vi "Find_Max_Value.vi"(3 "Mode":T6, 5 "Traverse line In":T1 {"Row Duration (mins)" format="%#.1f"; "Row No" min=0; "Trace Gas Concentration (%)" min=0.0 format="%#.2f"; "Emission Rate (l/min)" format="%#.2f"; "Tunnel Speed" format="%#.2f"; "Start X" format="%#.2f"; "Start Y" format="%#.2f"; "Start Z" format="%#.2f"; "End X" format="%#.2f"; "End Y" format="%#.2f"; "End Z" format="%#.2f"; "Averaging time (min)" min=0.0 format="%#.2f"}) -> (0 "Error Message":string, 1 "Status":T5, 2 "Traverse line Out":T1 {"Row Duration (mins)" format="%#.1f"; "Row No" min=0; "Trace Gas Concentration (%)" min=0.0 format="%#.2f"; "Emission Rate (l/min)" format="%#.2f"; "Tunnel Speed" format="%#.2f"; "Start X" format="%#.2f"; "Start Y" format="%#.2f"; "Start Z" format="%#.2f"; "End X" format="%#.2f"; "End Y" format="%#.2f"; "End Z" format="%#.2f"; "Averaging time (min)" min=0.0 format="%#.2f"})   [LabVIEW 2011]
uses:
  Controls/User_Specific_mode.ctl
  Gen Trav/Multi_Run_Status.ctl
  Gen Trav/Route mapping/Axis.ctl
  Gen Trav/Traverse_cluster.ctl
  Gen Trav/Spacing.ctl
  Controls/Multi_run_mode.ctl
  Controls/Tunnel_Coordinates.ctl
  Gen Trav/Trav_mode.ctl
  Controls/Save_Data.ctl
  Controls/Setup.ctl
  Globals/Meas_global.vi
panel:
  out "Measured Instrument":string
  out "Value to Measure":string
  in  "Channel to Measure":i32
  in  "Simulate?":bool
  in  "Picture Filename":path
  out "vi reference":refnum<vi>
  in  "Search Step (mm)":dbl=1.0
  out "Value at Maxima":dbl
  in  "Starting Position":dbl[](array[numeric]) format="%.1f"
  in  "stop":bool
  out "Message":string
  out "Y":i32
  out "X":i32
  out "Array 2":dbl[](array[numeric]) format="%.4f"
  out "Measured Points":dbl[][](array[numeric]) format="%.2f"
  out "Current Value":dbl format="%.2f"
  out "Current Index":i32
  out "Array":i32[][](array[numeric])
  out "Measurement":dbl[][](graph)
  out "Found Maxima?":bool
  out "Meas maxima":dbl[](array[numeric]) format="%.1f"
  out "Present Position":dbl[](array[numeric])
  out "Profile":dbl[][](array[numeric]) format="%.2f"
  in  "Fixed Axis":T4
  # "X           Y            Z"
  # "Start"
  # "End"
  # "X           Y            Z"
  # "Start"
  # "End"
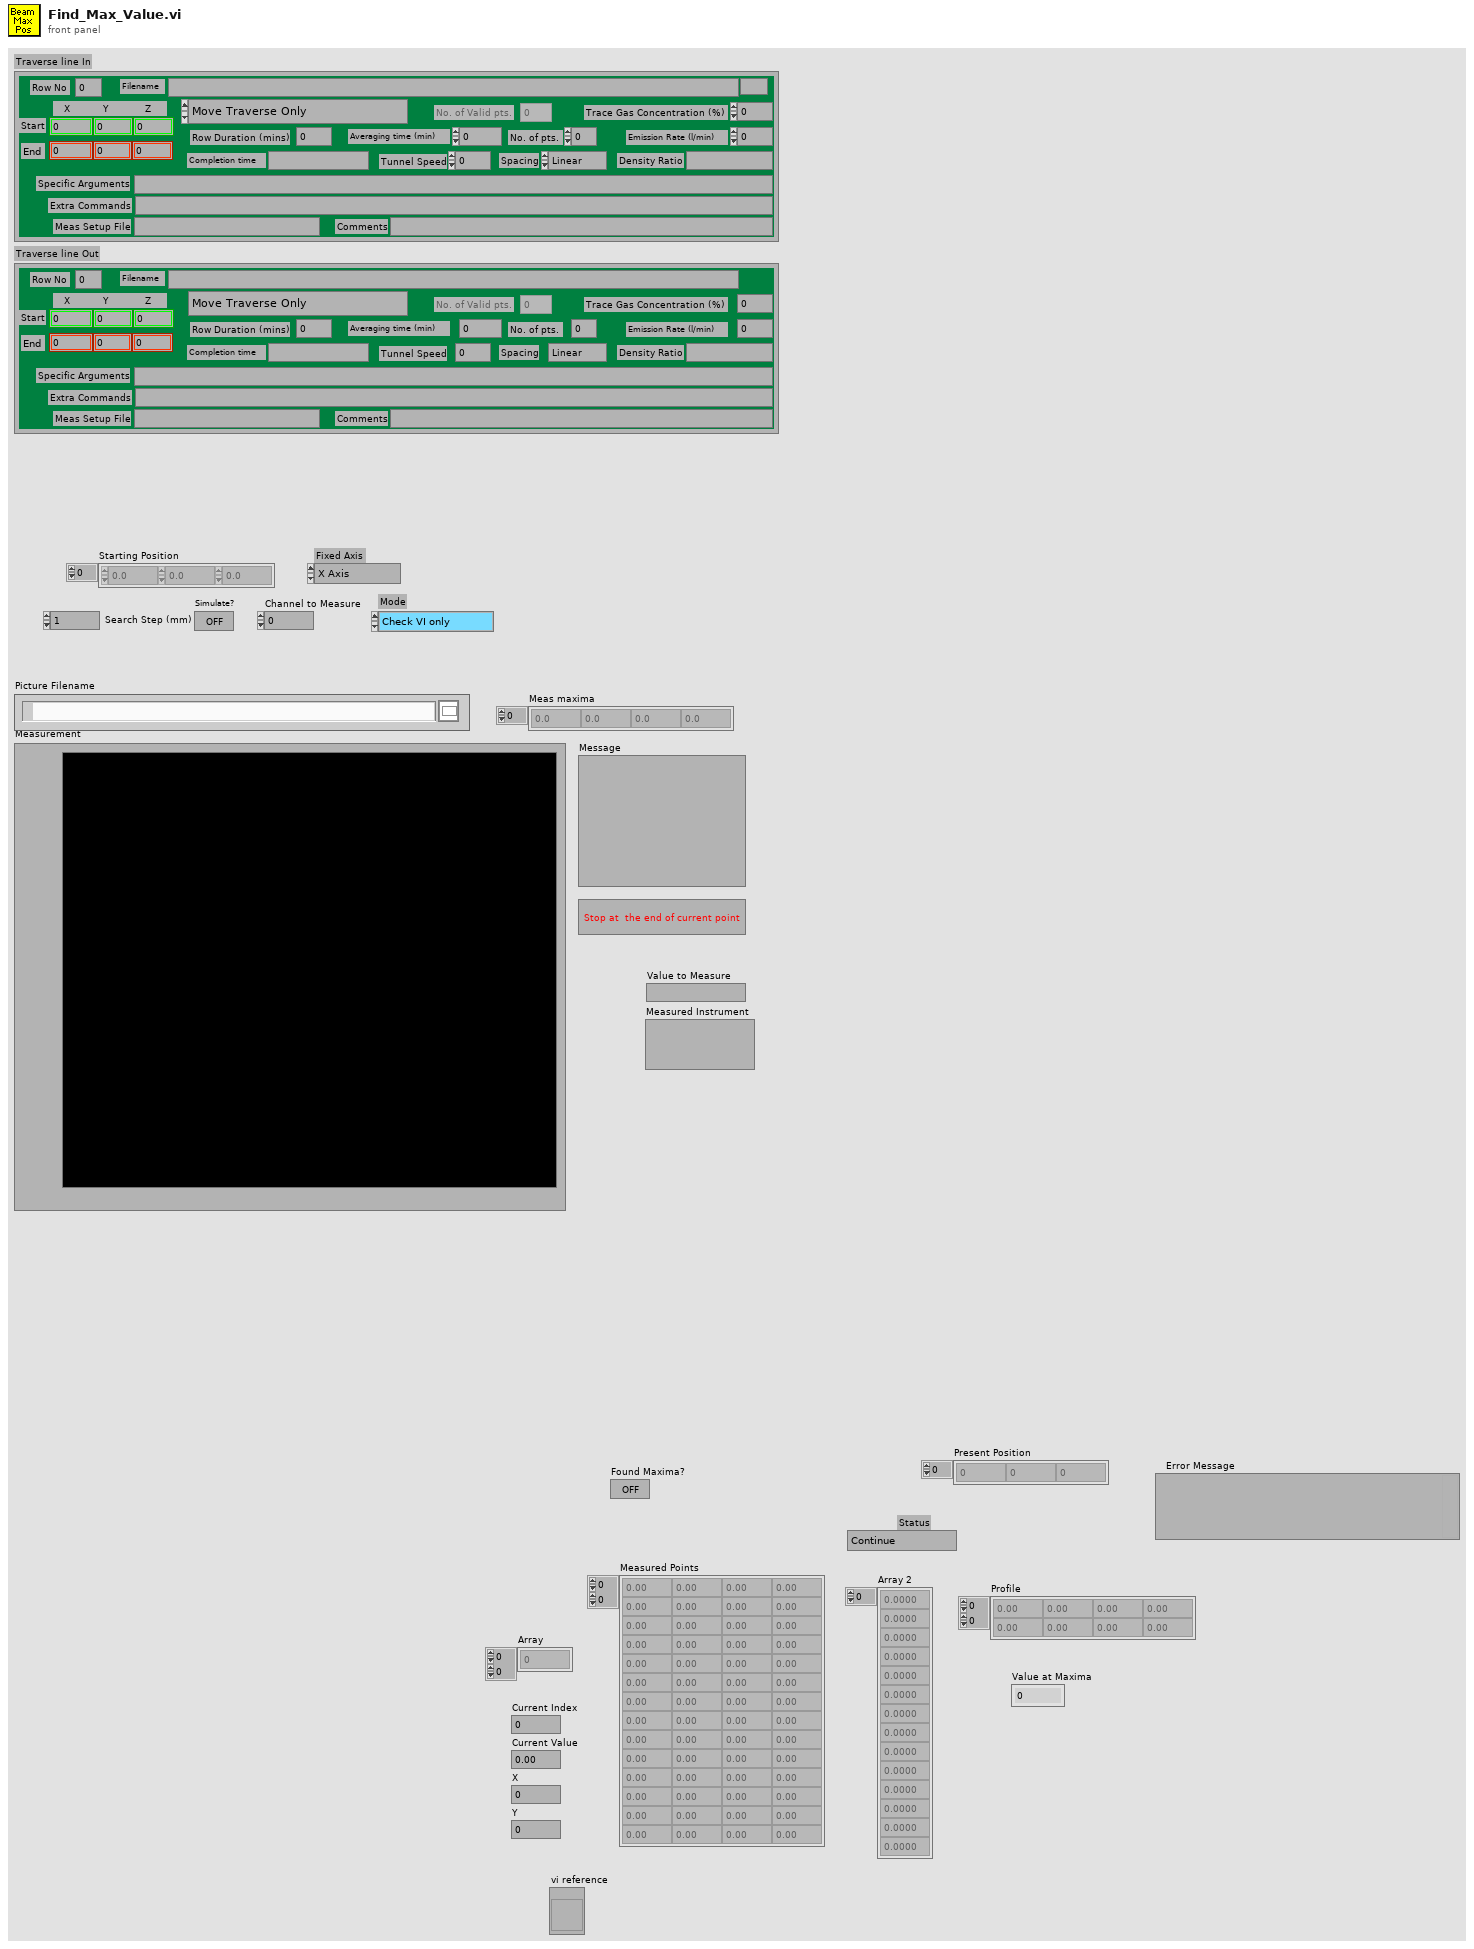
[diagram p1: front panel]
types:
  T1 = typedef "Traverse_cluster.ctl" = cluster{"Start X":dbl, "Start Y":dbl, "Start Z":dbl, "End X":dbl, "End Y":dbl, "End Z":dbl, "No. of pts.":i32, "Spacing":T2, "Filename":path, "Tunnel Speed":dbl, "Averaging time (min)":dbl, "Extra Commands":string, "Specific Arguments":string, "Emission Rate (l/min)":dbl, "Trace Gas Concentration (%)":dbl, "Density Ratio":string, "Comments":string, "Row No":i32, "Row Type Selector":T3, "Completion time":string, "Row Duration (mins)":dbl, "No. of Valid pts.":i32, "Meas Setup File":string}
  T2 = typedef "Spacing.ctl" = enum16{"Linear", "Log", "Gauss", "Specified", "N/A"}
  T3 = typedef "Multi_run_mode.ctl" = enum16{"Move Traverse Only", "Set Tunnel Speed Only", "Set Source Only", "Set Measurement Conditions", "Single Measurement", "Vertical Profile", "Lateral Profile", "Longitudinal Profile", "Explore Volume", "Multi-Axis Profile", "Auto Calibrate", "Meas Fast FID Bkgnd", "Check Beam Power", "Scanning Valve Measurement", "Run VI Named:", "Set ADAM Ch", "Wait (minutes)", "Send Message", "Synchronize With:", "Fall Back to this Row", "Turn Off Row Repeating", "Blank Row", "Traverse 3D Volume"}
  T4 = typedef "Axis.ctl" = enum16{"X Axis", "X Axis -ve", "Y Axis", "Y Axis -ve", "Z Axis", "Z Axis -ve"}
  T5 = typedef "Multi_Run_Status.ctl" = enum16{"Continue", "Jump to Next Point", "Jump to Next Row", "Jump To Fall Back", "Terminate Run"}
  T6 = typedef "User_Specific_mode.ctl" = enum16{"Check VI only", "Run VI"}
  T7 = typedef "Tunnel_Coordinates.ctl" = enum16{"Work in Tunnel Coordinates", "Work in Model Coordinates"}
  T8 = typedef "Trav_mode.ctl" = enum16{"Move traverse", "Read traverse position", "Teach Position"}
  T9 = cluster{"Status":enum16{"Continue", "Jump to Next Point", "Jump to Next Row", "Jump To Fall Back", "Terminate Run"}, "Error Type":string, "Error Description":string}
  T10 = typedef "Save_Data.ctl" = enum16{"Save No Data", "Save Data"}
  T11 = typedef "Setup.ctl" = enum16{"Run Program", "Show Setup", "Save Current Setup", "Setup Front Panel"}
  T12 = typedef "Status_Cluster.ctl" = cluster{"Status":T5, "Error Type":string, "Error Description":string}
  T13 = typedef "Analysis_info_cluster.ctl" = cluster{"Colour":u32, "Inst type":T14, "Inst name":string, "Symbol":string, "Code name":string, "Extra Info":string, "Inst Array":T15, "Extra Titles":string[], "Extra Values":string[], "U":dbl, "u^2":dbl, "u^3":dbl, "u^4":dbl, "Skew_u":dbl, "Kurt_u":dbl, "Sd Error in Mean":dbl, "% u'/U":dbl, "X":dbl, "Y":dbl, "Z":dbl, "Timescale integral to 25%":dbl, "Sd Error in Variance":dbl, "Calib File":path, "Calib Constants":dbl[], "Output Position":bool, "Full Stats":bool, "Av Sampling Rate":dbl, "Av No of Samples":dbl, "Total Meas Time (s)":dbl, "ADAM Ch Name":string}
  T14 = typedef "Inst_type.ctl" = enum16{"Propeller anemometer", "Raw voltage", "Pressure Transducer", "Pitot-static tube", "Preston tube", "Hot wire", "Cross wire 1", "Cross wire 2", "Generic Linear", "Generic Polynomial", "Generic BackPoly", "Fast FID", "Thermocouple", "Cold wire", "Pulsed Wire", "LDA Vel", "LDA Tran time", "LDA Arr time"}
  T15 = typedef "Instrument_Array.ctl" = enum16{"PWA", "LDA", "Analogue"}
  T16 = typedef "Correlation_cluster1.ctl" = cluster{"U inst":string, "uw":dbl, "u^2w":dbl, "uw^2":dbl, "uw/u'w'":dbl, "W inst":string, "uw^3":dbl, "u^3w":dbl, "u^2w^2":dbl, "Index U":i32, "Index W":i32}
  T17 = typedef "LVRectTypeDef.ctl" = cluster{"left":i16, "top":i16, "right":i16, "bottom":i16}
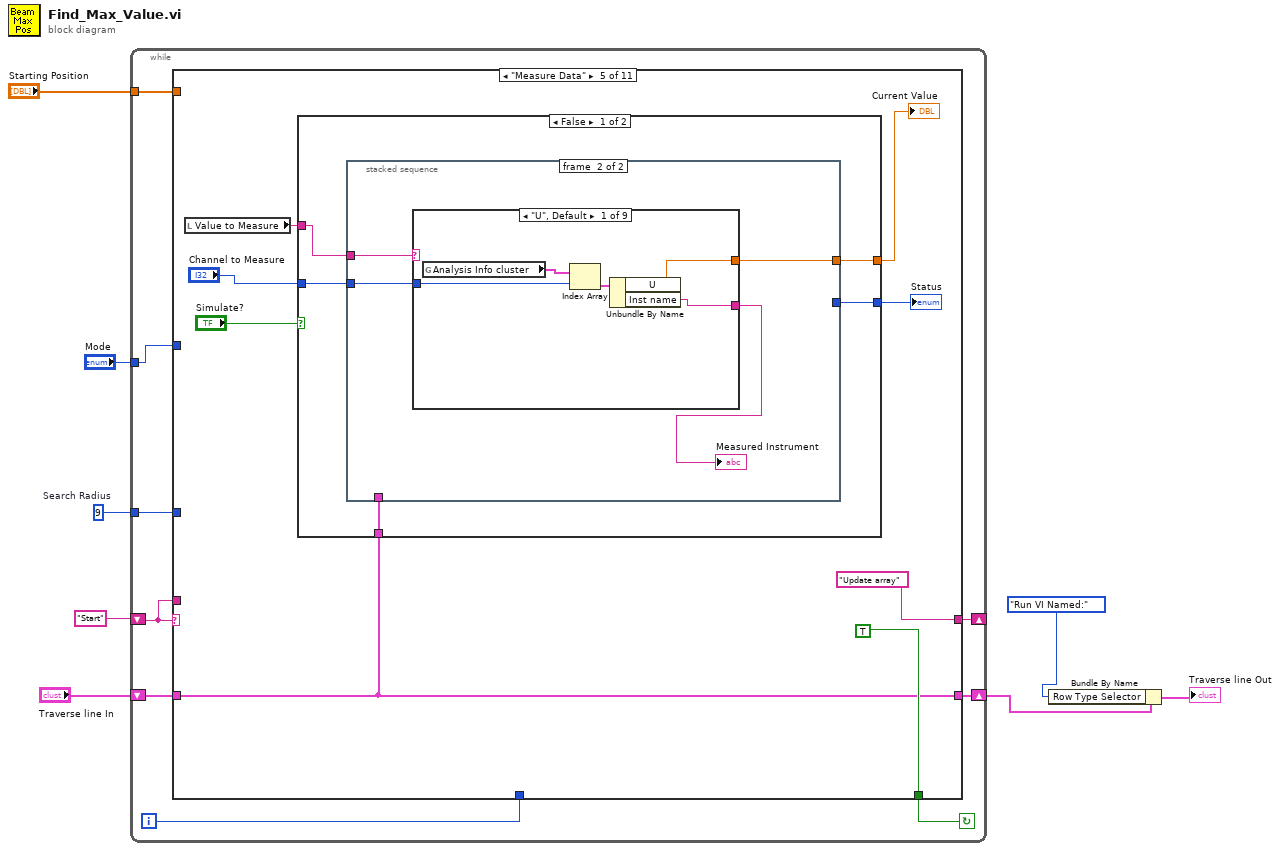
[diagram p0: block diagram]
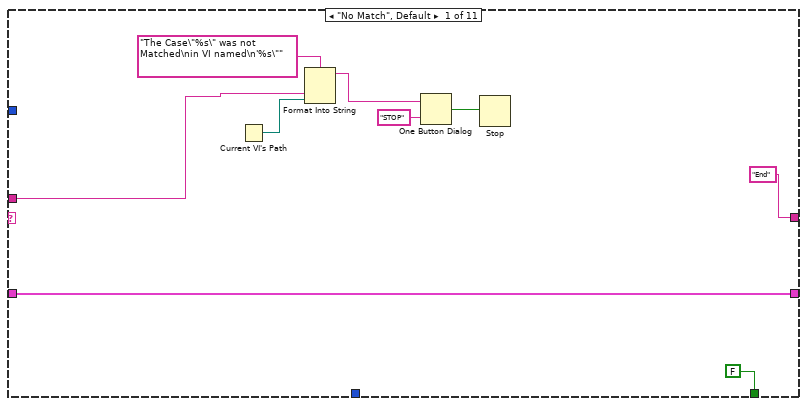
[diagram p2: hidden frame]
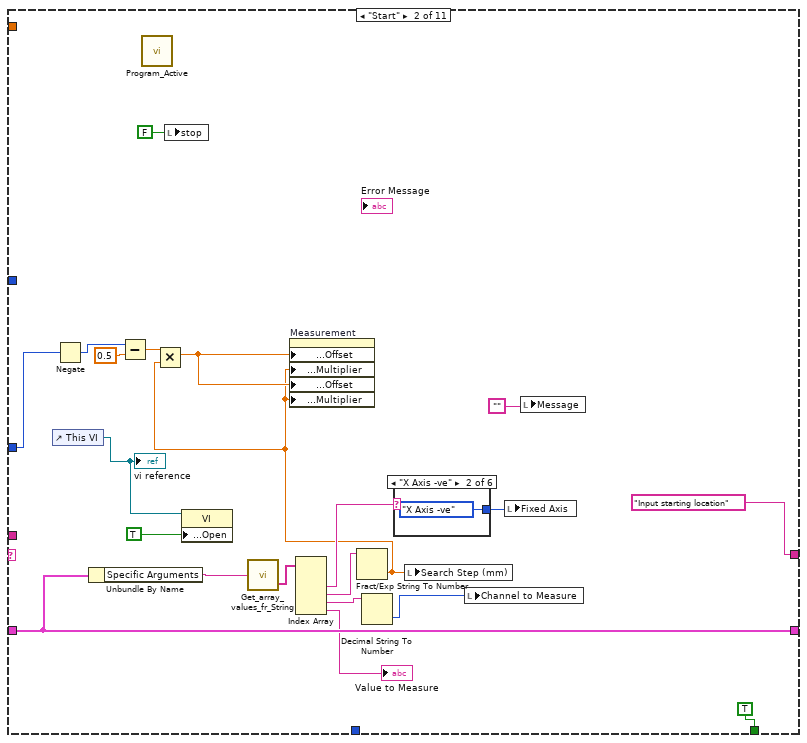
[diagram p3: hidden frame]
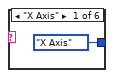
[diagram p4: hidden frame]
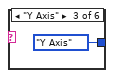
[diagram p5: hidden frame]
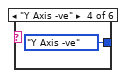
[diagram p6: hidden frame]
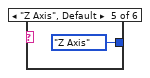
[diagram p7: hidden frame]
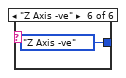
[diagram p8: hidden frame]
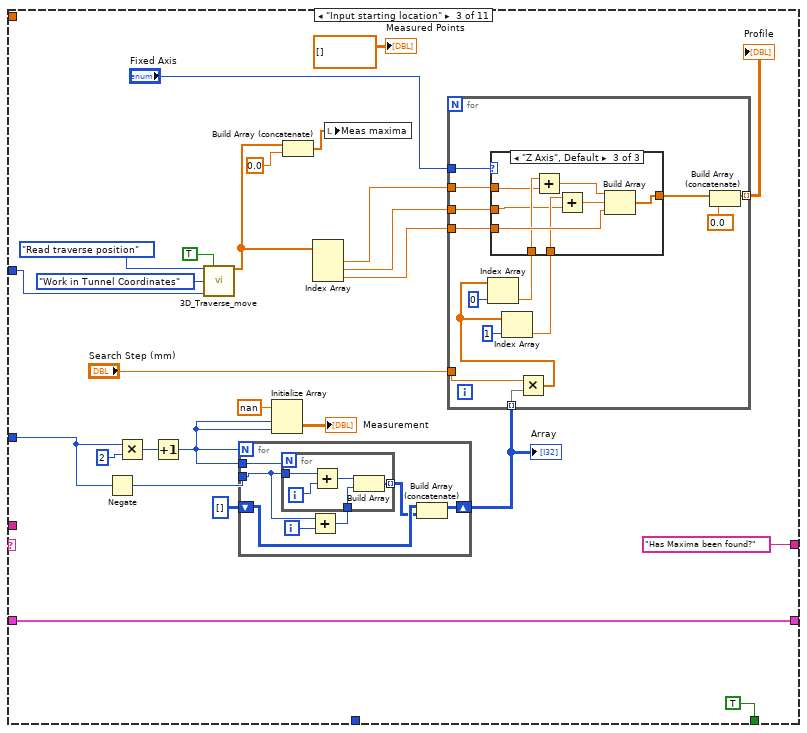
[diagram p9: hidden frame]
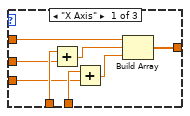
[diagram p10: hidden frame]
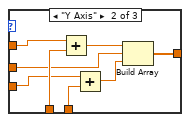
[diagram p11: hidden frame]
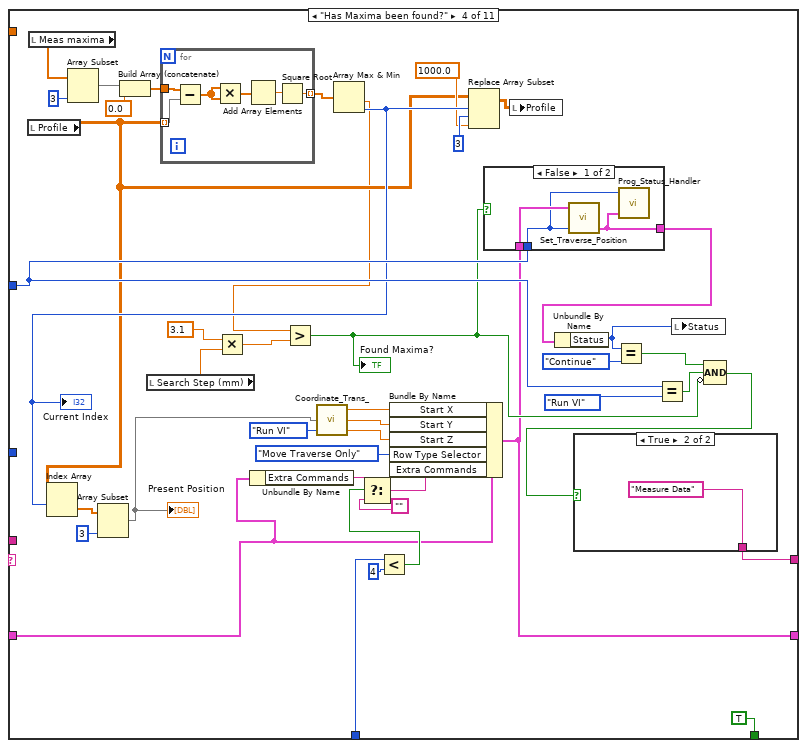
[diagram p12: hidden frame]
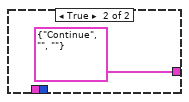
[diagram p13: hidden frame]
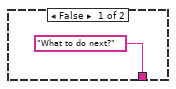
[diagram p14: hidden frame]
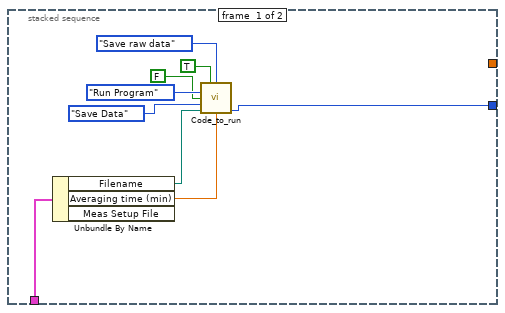
[diagram p15: hidden frame]
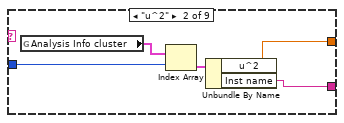
[diagram p16: hidden frame]
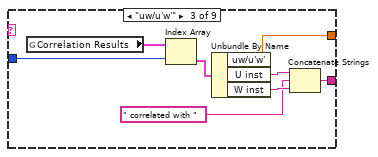
[diagram p17: hidden frame]
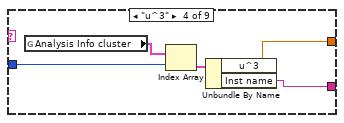
[diagram p18: hidden frame]
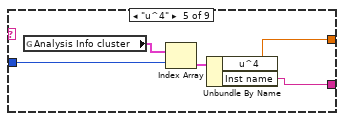
[diagram p19: hidden frame]
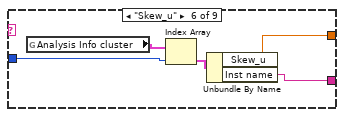
[diagram p20: hidden frame]
diagram:
  w7 = 9  # Search Radius
  n1 = while {
    tunnel: "Mode" -> [w15]
    shift-left: "Start" -> [w11]
    shift-right: [w16] -> _
    tunnel: w7 -> [w14]
    tunnel: "Starting Position" -> [w13]
    shift-right: [w9] -> w2
    shift-left: "Traverse line In" -> [w10]
    i -> [w12]
    stop <- w17 continue-if-true
    n2 = case shown="\"Measure Data\"" w11 {
      tunnel: w15 -> [_ _ w62 w167 _ _ _ w335 _ _ _]
      tunnel: [FALSE TRUE TRUE TRUE TRUE TRUE TRUE w329 TRUE TRUE FALSE] -> w17
      tunnel: ["End" "Input starting location" "Has Maxima been found?" w148 "Update array" "Calculate new maxima position" "What to do next?" w332 "Log Front Panel" "Get Interp Location" "End"] -> w16
      tunnel: w14 -> [_ w44 w69 _ _ w269 w289 _ _ _ _]
      tunnel: w13 -> [_ _ _ _ _ _ _ _ w355 _ _]
      tunnel: w12 -> [_ _ _ w134 _ _ _ _ _ _ _]
      tunnel: w11 -> [w21 _ _ _ _ _ _ _ _ _ _]
      tunnel: w10 -> [w18 w36 w64 w132 w186 w264 w282 w328 w343 w402 w417]
      tunnel: [w18 w36 w64 w131 w186 w264 w282 w328 w343 w402 w417] -> w9
      frame "No Match", Default {
        n3 = Current VI's Path() -> (path=w26:path)
        n4 = Format Into String(format string="The Case\"%s\" was not Matched\nin VI named\n'%s\"" ("Format String"), w21, w26) -> (resulting string=w23:string)  [unwired: 2 in, 1 out]
        n5 = One Button Dialog(message=w23, button name ("OK")="STOP") -> (true=w25:bool)
        n6 = Stop(stop? (T)=w25) -> ()
      }
      frame "Start" {
        n7 = control-ref of="This VI"() -> (w37:refnum<vi>)
        "vi reference" <- w37
        n8 = Negate(x=w44) -> (-x=w41:i32)
        n9 = Unbundle By Name(w36) -> ("Specific Arguments"=w35:string)
        n10 = Subtract(x=w41, y=0.5) -> (x-y=w42:dbl)
        n11 = call "Program_Active.vi"() -> ()  [unwired: 1 in]
        n12 = local write "stop"(FALSE ("stop")) -> ()
        n13 = property class="VI"(reference=w37, "Front Panel Window:Open"=TRUE) -> ()  [unwired: 1 in, 2 out]
        n14 = call "Get_array_values_fr_String.vi"("String Value"=w35) -> ("String array"=w34:string[])  [unwired: 1 out]
        n15 = Index Array(array=w34) -> (element #2=w33:string, element #3=w31:string, element #4=w29:string, element #5=→"Value to Measure":string)  [unwired: 5 in, 1 out]
        n16 = Fract/Exp String To Number(string=w31) -> (number=w30:dbl)  [unwired: 3 in, 1 out]
        n17 = Multiply(x=w42, y=w30) -> (x*y=w43:dbl)
        n18 = property on="Measurement" class="IntGraph (strict)"("X Scale.Offset and Multiplier:Offset"=w43, "X Scale.Offset and Multiplier:Multiplier"=w30, "Y Scale.Offset and Multiplier:Offset"=w43, "Y Scale.Offset and Multiplier:Multiplier"=w30) -> ()  [unwired: 2 in, 2 out]
        n19 = Decimal String To Number(string=w29) -> (number=w28:i32)  [unwired: 2 in, 1 out]
        n20 = case shown="\"X Axis -ve\"" w33 {
          tunnel: [Axis."X Axis" ("Fixed Axis") Axis."X Axis -ve" ("Fixed Axis") Axis."Y Axis" ("Fixed Axis") Axis."Y Axis -ve" ("Fixed Axis") Axis."Z Axis" ("Fixed Axis") Axis."Z Axis -ve" ("Fixed Axis")] -> w32
          frame "X Axis" {
          }
          frame "X Axis -ve" {
          }
          frame "Y Axis" {
          }
          frame "Y Axis -ve" {
          }
          frame "Z Axis", Default {
          }
          frame "Z Axis -ve" {
          }
        }
        n21 = local write "Search Step (mm)"(w30) -> ()
        n22 = local write "Channel to Measure"(w28) -> ()
        n23 = local write "Fixed Axis"(w32) -> ()
        n24 = local write "Message"("") -> ()
      }
      frame "Input starting location" {
        n25 = Negate(x=w69) -> (-x=w70:i32)
        n26 = Multiply(x=w69, y=2) -> (x*y=w67:i32)
        n27 = Increment(x=w67) -> (x+1=w66:i32)
        n28 = call "3D_Traverse_move.vi"("Mode"=Trav_mode."Read traverse position", "Route Checking?"=TRUE, "Work in Tunnel Coordinates"=Tunnel_Coordinates."Work in Tunnel Coordinates", "Simulate/Run"=w62) -> ("Trav Position achieved"=w59:dbl[])  [unwired: 9 in, 2 out]
        n29 = for {
          N: w66 -> [_]
          tunnel: w66 -> [w86]
          tunnel: w70 -> [w84]
          shift-right: [w80] -> w74
          shift-left: i32[][] [] -> [w82]
          i -> [w85]
          n30 = Add(x=w84, y=w85) -> (x+y=w83:i32)
          n31 = for {
            N: w86 -> [_]
            tunnel: w84 -> [w90]
            tunnel: w83 -> [w88]
            tunnel: [w87] -> w81 mode=indexing
            i -> [w91]
            n32 = Add(x=w90, y=w91) -> (x+y=w89:i32)
            n33 = Build Array(w89, w88) -> (w87:i32[])
          }
          n34 = Build Array (concatenate)(w82, w81) -> (w80:i32[][])
        }
        "Array" <- w74
        n35 = Initialize Array(nan, w66, w66) -> (→"Measurement":dbl[][])
        n36 = Build Array (concatenate)(w59, 0.0 ("Numeric")) -> (w76:dbl[])
        n37 = Index Array(array=w59) -> (element #1=w56:dbl, element #2=w57:dbl, element #3=w58:dbl)  [unwired: 3 in]
        n38 = local write "Meas maxima"(w76) -> ()
        n39 = for {
          tunnel: "Search Step (mm)" -> [w105]
          tunnel: w74 -> [w104] mode=indexing
          tunnel: "Fixed Axis" -> [w103]
          tunnel: w56 -> [w99]
          tunnel: w57 -> [w96]
          tunnel: w58 -> [w95]
          tunnel: [w93] -> w78 mode=indexing
          n40 = Multiply(x=w105, y=w104) -> (x*y=w100:dbl[])
          n41 = Index Array(array=w100, index=0 ("Index")) -> (element=w98:dbl)
          n42 = Index Array(array=w100, index=1 ("Index")) -> (element=w97:dbl)
          n43 = case shown="\"Z Axis\", Default" w103 {
            tunnel: w99 -> [w113 w120 w124]
            tunnel: w98 -> [w112 w118 w127]
            tunnel: w97 -> [w111 w117 w126]
            tunnel: w96 -> [w110 w114 w125]
            tunnel: w95 -> [w109 w116 w128]
            tunnel: [w106 w121 w129] -> w94
            frame "X Axis" {
              n44 = Add(x=w112, y=w110) -> (x+y=w108:dbl)
              n45 = Add(x=w111, y=w109) -> (x+y=w107:dbl)
              n46 = Build Array(w113, w108, w107) -> (w106:dbl[])
            }
            frame "Y Axis" {
              n47 = Add(x=w120, y=w118) -> (x+y=w119:dbl)
              n48 = Add(x=w116, y=w117) -> (x+y=w115:dbl)
              n49 = Build Array(w119, w114, w115) -> (w121:dbl[])
            }
            frame "Z Axis", Default {
              n50 = Add(x=w127, y=w124) -> (x+y=w123:dbl)
              n51 = Add(x=w126, y=w125) -> (x+y=w122:dbl)
              n52 = Build Array(w123, w122, w128) -> (w129:dbl[])
            }
          }
          n53 = Build Array (concatenate)(w94, 0.0 ("Input Element")) -> (w93:dbl[])
        }
        "Profile" <- w78
        "Measured Points" <- dbl[][] [] ("Measured Points")
      }
      frame "Has Maxima been found?" {
        n54 = local read "Profile"() -> (w154:dbl[][])
        n55 = local read "Meas maxima"() -> (w164:dbl[])
        n56 = Array Subset(array=w164, length=3 ("Array Length")) -> (w161:dbl[])  [unwired: 1 in]
        n57 = Build Array (concatenate)(w161, 0.0 ("Input Element")) -> (w160:dbl[])
        n58 = local read "Search Step (mm)"() -> (w130:dbl)
        n59 = for {
          tunnel: w154 -> [w183] mode=indexing
          tunnel: w160 -> [w182]
          tunnel: [w178] -> w162 mode=indexing
          n60 = Subtract(x=w182, y=w183) -> (x-y=w180:dbl[])
          n61 = Multiply(x=w180, y=w180) -> (x*y=w179:dbl[])
          n62 = Add Array Elements(numeric array=w179) -> (sum=w181:dbl)
          n63 = Square Root(x=w181) -> (sqrt(x)=w178:dbl)
        }
        n64 = Multiply(x=3.1, y=w130) -> (x*y=w151:dbl)
        n65 = Unbundle By Name(w132) -> ("Extra Commands"=w146:string)
        n66 = Array Max & Min(array=w162) -> (min value=w152:dbl, min index (indices)=w158:i32)  [unwired: 2 out]
        "Current Index" <- w158
        n67 = Index Array(array=w154, index (row)=w158) -> (element=w137:dbl[])  [unwired: 1 in]
        n68 = Array Subset(array=w137, length=3) -> (w136:dbl[])  [unwired: 1 in]
        "Present Position" <- w136
        n69 = Greater?(x=w152, y=w151) -> (0:w141:bool)
        "Found Maxima?" <- w141
        n70 = call "Coordinate_Trans_.vi"("Simulate/Run"=User_Specific_mode."Run VI", "Input Position"=w136) -> ("Z"=w140:dbl, "Y"=w139:dbl, "X"=w138:dbl)  [unwired: 1 in]
        n71 = Less?(x=w134, y=4) -> (x < y?=w144:bool)
        n72 = Select(t=w146, s=w144, f="") -> (s? t:f=w142:string)
        n73 = Bundle By Name(cluster=w132, "Start X"=w138, "Start Y"=w139, "Start Z"=w140, "Row Type Selector"=Multi_run_mode."Move Traverse Only", "Extra Commands"=w142) -> (w131:T1)
        n74 = Replace Array Subset(array=w154, new element=1000.0 ("Element Data"), index (row)=w158, index (col)=3 ("Index")) -> (w155:dbl[][])
        n75 = case shown="False" w141 {
          tunnel: [w173 T9 {"Status"=enum."Continue", "Error Type"="", "Error Description"=""} ("Status Cluster")] -> w169
          tunnel: w167 -> [w172 _]
          tunnel: w131 -> [w174 _]
          frame False {
            n76 = call "Set_Traverse_Position.vi"("Simulate/Run"=w172, "Traverse line"=w174) -> ("Status Cluster"=w173:T12)  [unwired: 1 in, 2 out]
            n77 = call "Prog_Status_Handler.vi"("Status Cluster"=w173, "Simulate/Run"=w172) -> ()  [unwired: 2 out]
          }
          frame True {
          }
        }
        n78 = local write "Profile"(w155) -> ()
        n79 = Unbundle By Name(w169) -> ("Status"=w165:T5)
        n80 = Equal?(x=w165, y=Multi_Run_Status."Continue" ("Status")) -> (x = y?=w150:bool)
        n81 = Equal?(x=w167, y=User_Specific_mode."Run VI" ("Mode")) -> (x = y?=w149:bool)
        n82 = local write "Status"(w165) -> ()
        n83 = Compound Arithmetic op=AND(w150, w149, invert w141) -> (w147:bool)
        n84 = case shown="True" w147 {
          tunnel: ["What to do next?" "Measure Data"] -> w148
          frame False {
          }
          frame True {
          }
        }
      }
      frame "Measure Data" {
        n85 = local read "Value to Measure"() -> (w184:string)
        n86 = case shown="False" "Simulate?" {
          tunnel: [w195 w260] -> w189
          tunnel: [w194 w262] -> w188
          tunnel: w186 -> [w196 _]
          tunnel: "Channel to Measure" -> [w193 _]
          tunnel: w184 -> [w192 _]
          frame False {
            n87 = stacked-sequence {
              tunnel: w196 -> [w200 _]
              tunnel: [w197 _] -> w195
              tunnel: [_ w208] -> w194
              tunnel: w193 -> [_ w207]
              tunnel: w192 -> [_ w209]
              frame #0 {
                n88 = Unbundle By Name(w200) -> ("Filename"=w198:path, "Averaging time (min)"=w199:dbl)  [unwired: 1 out]
                n89 = call "Code_to_run.vi"("Open Front Panel"=TRUE, "Raw data option"=enum16{"Save raw data", "Raw data not saved"}."Save raw data", "setup"=Setup."Run Program", "Remote control"=FALSE, "File"=Save_Data."Save Data", "Results Filename"=w198, "Averaging time (min)"=w199) -> ("Status"=w197:T5)  [unwired: 4 in, 4 out]
              }
              frame #1 {
                n90 = case shown="\"U\", Default" w209 {
                  tunnel: [w212 w217 w226 w230 w235 w240 w245 w250 w255] -> w208
                  tunnel: w207 -> [w211 w216 w225 w229 w234 w239 w244 w249 w254]
                  tunnel: [w210 w215 w220 w228 w233 w238 w243 w248 w253] -> w206
                  frame "U", Default {
                    n91 = global read "Meas_global.vi" "Analysis Info cluster"() -> (w213:T13[])
                    n92 = Index Array(array=w213, index=w211) -> (element=w214:T13)
                    n93 = Unbundle By Name(w214) -> ("U"=w212:dbl, "Inst name"=w210:string)
                  }
                  frame "u^2" {
                    n94 = global read "Meas_global.vi" "Analysis Info cluster"() -> (w218:T13[])
                    n95 = Index Array(array=w218, index=w216) -> (element=w219:T13)
                    n96 = Unbundle By Name(w219) -> ("u^2"=w217:dbl, "Inst name"=w215:string)
                  }
                  frame "uw/u'w'" {
                    n97 = global read "Meas_global.vi" "Correlation Results"() -> (w224:T16[])
                    n98 = Index Array(array=w224, index=w225) -> (element=w227:T16)
                    n99 = Unbundle By Name(w227) -> ("uw/u'w'"=w226:dbl, "U inst"=w223:string, "W inst"=w222:string)
                    n100 = Concatenate Strings(w223, " correlated with " ("string"), w222) -> (w220:string)
                  }
                  frame "u^3" {
                    n101 = global read "Meas_global.vi" "Analysis Info cluster"() -> (w231:T13[])
                    n102 = Index Array(array=w231, index=w229) -> (element=w232:T13)
                    n103 = Unbundle By Name(w232) -> ("u^3"=w230:dbl, "Inst name"=w228:string)
                  }
                  frame "u^4" {
                    n104 = global read "Meas_global.vi" "Analysis Info cluster"() -> (w236:T13[])
                    n105 = Index Array(array=w236, index=w234) -> (element=w237:T13)
                    n106 = Unbundle By Name(w237) -> ("u^4"=w235:dbl, "Inst name"=w233:string)
                  }
                  frame "Skew_u" {
                    n107 = global read "Meas_global.vi" "Analysis Info cluster"() -> (w241:T13[])
                    n108 = Index Array(array=w241, index=w239) -> (element=w242:T13)
                    n109 = Unbundle By Name(w242) -> ("Skew_u"=w240:dbl, "Inst name"=w238:string)
                  }
                  frame "Kurt_u" {
                    n110 = global read "Meas_global.vi" "Analysis Info cluster"() -> (w246:T13[])
                    n111 = Index Array(array=w246, index=w244) -> (element=w247:T13)
                    n112 = Unbundle By Name(w247) -> ("Kurt_u"=w245:dbl, "Inst name"=w243:string)
                  }
                  frame "% u'/U" {
                    n113 = global read "Meas_global.vi" "Analysis Info cluster"() -> (w251:T13[])
                    n114 = Index Array(array=w251, index=w249) -> (element=w252:T13)
                    n115 = Unbundle By Name(w252) -> ("% u'/U"=w250:dbl, "Inst name"=w248:string)
                  }
                  frame "Sd Error in Mean" {
                    n116 = global read "Meas_global.vi" "Analysis Info cluster"() -> (w256:T13[])
                    n117 = Index Array(array=w256, index=w254) -> (element=w257:T13)
                    n118 = Unbundle By Name(w257) -> ("Sd Error in Mean"=w255:dbl, "Inst name"=w253:string)
                  }
                }
                "Measured Instrument" <- w206
              }
            }
          }
          frame True {
            n119 = call "Input_Value_Dialog.vi"("Message to user"="Enter Test Value") -> ("Value received"=w262:dbl, "Ok Out"=w261:bool)
            n120 = Select(t=Multi_Run_Status."Continue" ("Status"), s=w261, f=Multi_Run_Status."Terminate Run" ("Status")) -> (s? t:f=w260:T5)
          }
        }
        "Current Value" <- w188
        "Status" <- w189
      }
      frame "Update array" {
        w266 = TRUE ("Front Panel Window:Open")
        n121 = local read "Current Index"() -> (w279:i32)
        n122 = local read "vi reference"() -> (w267:refnum<vi>)
        n123 = local read "Array"() -> (w278:i32[][])
        n124 = property class="VI"(reference=w267, "Front Panel Window:Open"=w266, "Front Panel Window:Auto Center (Deprecated)"=w266) -> ()  [unwired: 1 in, 2 out]
        n125 = Index Array(array=w278, index (row)=w279, index (col)=1 ("Index")) -> (element=w273:i32)
        n126 = Index Array(array=w278, index (row)=w279, index (col)=0 ("Index")) -> (element=w272:i32)
        n127 = local read "Measurement"() -> (w275:dbl[][])
        n128 = local read "Current Value"() -> (w265:dbl)
        n129 = Add(x=w273, y=w269) -> (x+y=w270:i32)
        "Y" <- w270
        n130 = Add(x=w272, y=w269) -> (x+y=w271:i32)
        "X" <- w271
        n131 = Replace Array Subset(array=w275, new element=w265, index (row)=w271, index (col)=w270) -> (w274:dbl[][])
        n132 = local write "Measurement"(w274) -> ()
      }
      frame "Calculate new maxima position" {
        n133 = local read "Present Position"() -> (w304:dbl[])
        n134 = local read "Measured Points"() -> (w305:dbl[][])
        n135 = local read "Current Value"() -> (w303:dbl)
        n136 = local read "X"() -> (w298:i32)
        n137 = local read "Y"() -> (w297:i32)
        n138 = Negate(x=w289) -> (-x=w287:i32)
        n139 = Build Array (concatenate)(w304, w303, w298, w297) -> (w302:dbl[])
        n140 = local read "Search Step (mm)"() -> (w281:dbl)
        n141 = Build Array (concatenate)(w305, w302) -> (w299:dbl[][])
        n142 = for {
          tunnel: w299 -> [w314] mode=indexing
          tunnel: w299 -> [w312]
          tunnel: w281 -> [w310]
          tunnel: [w307] -> w301 mode=indexing
          n143 = Array Subset(array=w314, length=3 ("Array Length")) -> (w311:dbl[])  [unwired: 1 in]
          n144 = for {
            tunnel: w312 -> [w321] mode=indexing
            tunnel: w311 -> [w326]
            tunnel: w310 -> [w316]
            tunnel: [w318] -> w308 mode=indexing
            tunnel: [w315] -> w309 mode=indexing
            n145 = Array Subset(array=w321, length=3 ("Array Length")) -> (w325:dbl[])  [unwired: 1 in]
            n146 = Subtract(x=w326, y=w325) -> (x-y=w322:dbl[])
            n147 = Multiply(x=w322, y=w322) -> (x*y=w323:dbl[])
            n148 = Add Array Elements(numeric array=w323) -> (sum=w324:dbl)
            n149 = Square Root(x=w324) -> (sqrt(x)=w319:dbl)
            n150 = Add(x=w319, y=w316) -> (x+y=w317:dbl)
            n151 = Index Array(array=w321, index=3 ("Index")) -> (element=w315:dbl)
            n152 = Divide(x=w316, y=w317) -> (x/y=w318:dbl)
          }
          n153 = call "Weighted_Mean_fr_NaN_data.vi"("Weighting"=w308, "Data"=w309) -> ("Mean value"=w307:dbl)
        }
        "Array 2" <- w301
        n154 = local write "Measured Points"(w299) -> ()
        n155 = Array Max & Min(array=w301) -> (max index (indices)=w300:i32)  [unwired: 3 out]
        n156 = Index Array(array=w299, index (row)=w300) -> (element=w292:dbl[])  [unwired: 1 in]
        n157 = Index Array(array=w292, index=5 ("Index")) -> (element=w290:dbl)
        n158 = Array Subset(array=w292, length=4 ("Array Length")) -> (→"Meas maxima":dbl[])  [unwired: 1 in]
        n159 = Index Array(array=w292, index=4 ("Index")) -> (element=w291:dbl)
        n160 = Add(x=w287, y=w291) -> (x+y=w286:dbl)
        n161 = Add(x=w287, y=w290) -> (x+y=w285:dbl)
        n162 = Multiply(x=w281, y=w285) -> (x*y=w284:dbl)
        n163 = Multiply(x=w281, y=w286) -> (x*y=w283:dbl)
        n164 = property on="Intensity Graph" class="IntGraph (strict)"("Cursor.Cursor Position:Cursor X"=w283, "Cursor.Cursor Position:Cursor Y"=w284) -> ()  [unwired: 2 in, 2 out]
      }
      frame "What to do next?" {
        n165 = local read "Found Maxima?"() -> (w337:bool)
        n166 = case shown="False" "stop" {
          tunnel: [w339 w340] -> w333
          frame False {
            n167 = local read "Status"() -> (w339:T5)
          }
          frame True {
            w340 = Multi_Run_Status."Terminate Run" ("Status")
            n168 = local write "Status"(w340) -> ()
          }
        }
        n169 = case shown="False" w337 {
          tunnel: ["Has Maxima been found?" "Compile Message"] -> w332
          frame False {
          }
          frame True {
          }
        }
        n170 = Equal?(x=w335, y=User_Specific_mode."Run VI" ("Mode")) -> (x = y?=w331:bool)
        n171 = Equal?(x=w333, y=Multi_Run_Status."Continue" ("Status")) -> (x = y?=w330:bool)
        n172 = And(x=w330, y=w331) -> (x .and. y?=w329:bool)
      }
      frame "Compile Message" {
        # "X Y Z Data"
        n173 = local read "Meas maxima"() -> (w354:dbl[])
        n174 = Build Array("X", "Y", "Z", "Value" ("Input Element")) -> (w360:string[])
        n175 = Index Array(array=w354, index=3) -> (element=w352:dbl)
        n176 = call "Orb_Calibration.vi"("Voltage"=w352) -> ("Normalised Voltage"=w350:dbl)  [unwired: 1 out]
        "Value at Maxima" <- w350
        n177 = for {
          tunnel: w354 -> [w376] mode=indexing
          shift-right: [w374] -> w359
          shift-left: "" -> [w375]
          tunnel: w360 -> [w373] mode=indexing
          tunnel: [w372] -> w356 mode=indexing
          tunnel: w355 -> [w371]
          tunnel: w350 -> [w369]
          shift-right: [w367] -> w346
          shift-left: " Final Position " -> [w368]
          i -> [w370]
          n178 = case shown="0, Default" w370 {
            tunnel: w376 -> [w378 w399]
            tunnel: w375 -> [w388 w395]
            tunnel: [w387 w395] -> w374
            tunnel: w373 -> [w379 w401]
            tunnel: [w385 TRUE] -> w372
            tunnel: w371 -> [w384 _]
            tunnel: w370 -> [w383 _]
            tunnel: w369 -> [_ _]
            tunnel: w368 -> [w380 w397]
            tunnel: [w377 w396] -> w367
            frame 0, Default {
              n179 = Index Array(array=w384, index=w383) -> (element=w382:dbl)
              n180 = Subtract(x=w378, y=w382) -> (x-y=w386:dbl)
              n181 = Format Into String(format string="%s=%.1fmm, " ("Format String"), initial string=w380, w379, w378) -> (resulting string=w377:string)  [unwired: 1 in, 1 out]
              n182 = Equal To 0?(x=w386) -> (x = 0?=w385:bool)
              n183 = case shown="False" w385 {
                tunnel: w388 -> [w393 w394]
                tunnel: [w392 w394] -> w387
                tunnel: w379 -> [w391 _]
                tunnel: w386 -> [w389 _]
                frame False {
                  n184 = Format Into String(format string="%s=%.1fmm, " ("Format String"), initial string=w393, w391, w389) -> (resulting string=w392:string)  [unwired: 1 in, 1 out]
                }
                frame True {
                }
              }
            }
            frame 3 {
              n185 = Format Into String(format string="%s=%.3f" ("Format String"), initial string=w397, w401, w399) -> (resulting string=w396:string)  [unwired: 1 in, 1 out]
            }
          }
        }
        n186 = And Array Elements(Boolean array=w356) -> (logical AND=w349:bool)
        n187 = case shown="False" w349 {
          tunnel: ["Position Unchanged " ("Format String") "Position tweaked by " ("Format String")] -> w358
          frame True {
          }
          frame False {
          }
        }
        n188 = Concatenate Strings(w358, w359, w346, "\r\n") -> (→"Message":string)
      }
      frame "Log Front Panel" {
        n189 = Empty String/Path?(string/path="Picture Filename") -> (empty?=w406:bool)
        n190 = local read "vi reference"() -> (w404:refnum<vi>)
        n191 = case shown="False" w406 {
          tunnel: "Picture Filename" -> [w408 _]
          frame False {
            w414 = 24 ("image depth")
            n192 = control-ref of="This VI"() -> (w415:refnum<vi>)
            n193 = invoke class="VI" method="FP.Old Get Image"(reference=w415, "visible area only"=TRUE, "image depth"=w414) -> (error out=w410:errorcluster, "image"=w411:u8[], "colors"=w413:u32[], "bounds"=w412:T17)  [unwired: 5 in, 4 out]
            n194 = call <vilib>:"Write PNG File(6_1).vi"("color table"=w413, "depth"=w414, "error in (no error)"=w410, "flattened image data"=w411, "rect"=w412, "path to PNG file"=w408) -> ()  [unwired: 6 out]
          }
          frame True {
          }
        }
        n195 = Close Reference(reference=w404) -> ()  [unwired: 1 in, 1 out]
      }
      frame "Get Interp Location" {
        w418 = 3 items=["nearest", "bilinear", "bicubic", "bicubic spline"] ("method")
        n196 = local read "Fixed Axis"() -> (w416:T4)
        n197 = local read "Measured Points"() -> (w421:dbl[][])
        n198 = local read "Meas maxima"() -> (w420:dbl[])
        n199 = call "Interp2D.vi"("method"=w418, "Fixed Axis"=w416, "Interpolation Points"=100, "Meas maxima"=w420, "Measured Points"=w421) -> ()  [unwired: 4 in, 3 out]
      }
    }
  }
  n200 = Bundle By Name(cluster=w2, "Row Type Selector"=Multi_run_mode."Run VI Named:") -> (→"Traverse line Out":T1)
